vi "6.1_BuildString.vi"(4 "String 2":string="Volts DC: +1.26E+1", 5 "Trailer":string, 6 "Numeric":dbl, 7 "Header":string) -> (0 "Offset Past Match":i32, 1 "Number Out":dbl, 2 "String Length":i32, 3 "Combined String":string)   [LabVIEW 2025]
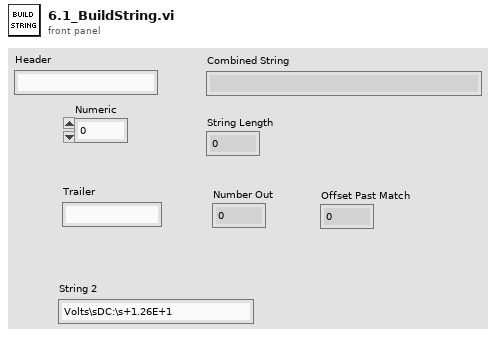
[diagram p1: front panel]
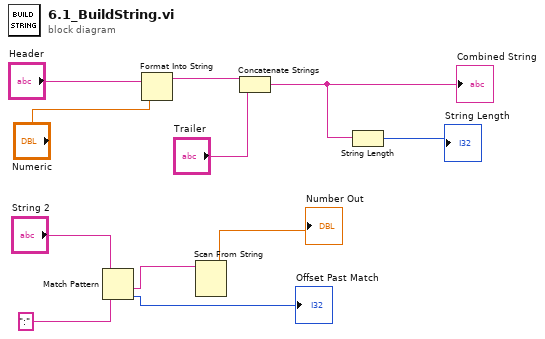
[diagram p0: block diagram]
diagram:
  n1 = Match Pattern(string=":", regular expression="String 2") -> (after substring=w3:string, offset past match=→"Offset Past Match":i32)  [unwired: 1 in, 2 out]
  n2 = Format Into String(initial string="Header", "Numeric") -> (resulting string=w9:string)  [unwired: 2 in, 1 out]
  n3 = Scan From String(input string=w3) -> (output 1=→"Number Out":dbl)  [unwired: 4 in, 3 out]
  n4 = Concatenate Strings(w9, "Trailer") -> (w6:string)
  "Combined String" <- w6
  n5 = String Length(string=w6) -> (length=→"String Length":i32)
